vi "appendImage.vi"(8 "error in (no error)":errorcluster, 10 "Image Path":path, 11 "MS-Excel in":refnum<class "MS-Excel.lvclass">) -> (0 "error out":errorcluster, 3 "MS-Excel out":refnum<class "MS-Excel.lvclass">)   [LabVIEW 2017, in "LabVIEW NPOI.lvlib" / "MS-Excel.lvclass"]
uses:
  MS-Excel.lvclass
  MS-Excel.lvclass/MS-Excel.ctl
  C:/Users/Neo/Desktop/Dev_Tools_BR/LabVIEW_NPOI/lib/NPOI 2.1.1/NPOI.dll
  lib/NPOI 2.1.1/NPOI.dll
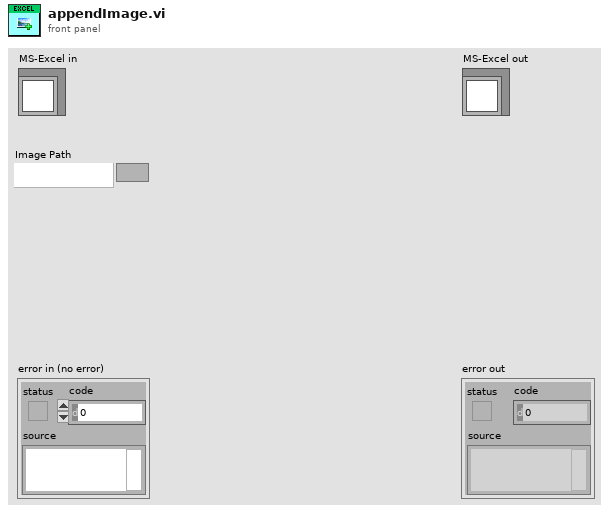
[diagram p1: front panel]
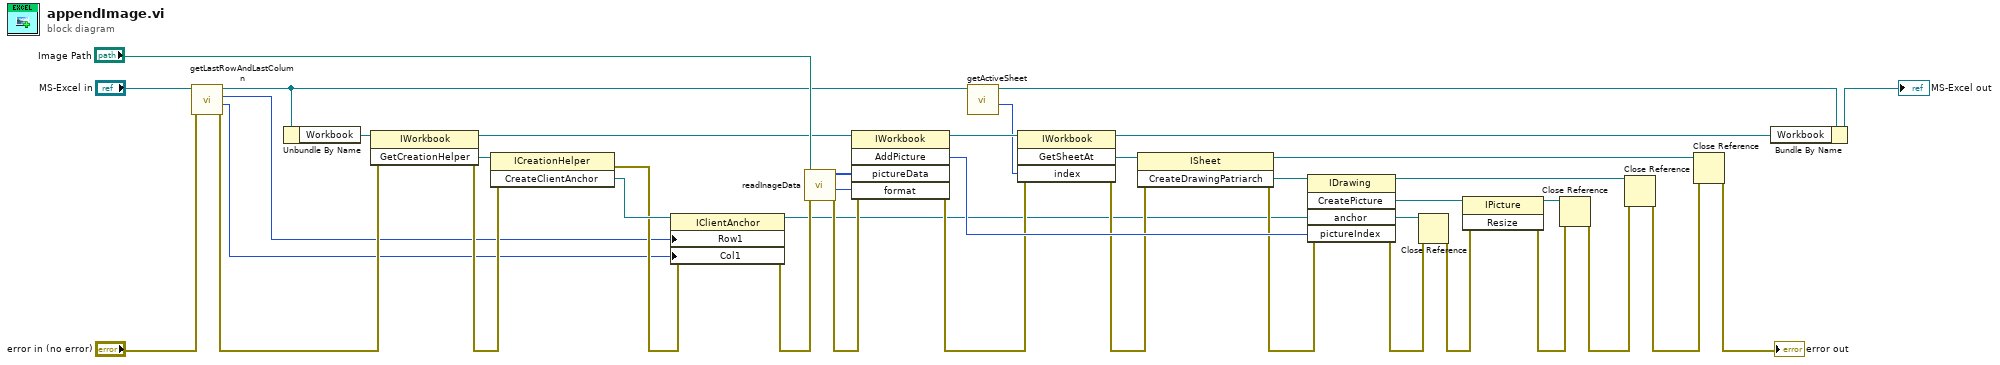
[diagram p0: block diagram]
diagram:
  n1 = call-dynamic "getLastRowAndLastColumn.vi"("error in (no error)"="error in (no error)", "MS-Excel in"="MS-Excel in") -> ("error out"=w23:errorcluster, "Last Column"=w1:i32, "Last Row"=w2:i32, "MS-Excel out"=w26:refnum<class "MS-Excel.lvclass">)  [unwired: 6 in]
  n2 = Unbundle By Name(w26) -> ("Workbook"=w24:refnum<k24>)
  n3 = invoke class="IWorkbook" method="GetCreationHelper"(reference=w24, error in=w23) -> (reference out=w18:refnum<k24>, error out=w22:errorcluster, "GetCreationHelper"=w38:refnum<k24>)  [unwired: 1 in]
  n4 = invoke class="ICreationHelper" method="CreateClientAnchor"(reference=w38, error in=w22) -> (error out=w3:errorcluster, "CreateClientAnchor"=w37:refnum<k24>)  [unwired: 1 in, 1 out]
  n5 = property class="IClientAnchor"(reference=w37, error in=w3, "Row1"=w2, "Col1"=w1) -> (reference out=w16:refnum<k24>, error out=w21:errorcluster)
  n6 = call "readInageData.vi"("error in (no error)"=w21, "file (use dialog)"="Image Path") -> ("error out"=w20:errorcluster, "format"=w28:i32, "Bytes"=w34:u8[])  [unwired: 7 in]
  n7 = invoke class="IWorkbook" method="AddPicture"(reference=w18, error in=w20, "pictureData"=w34, "format"=w28) -> (reference out=w17:refnum<k24>, error out=w19:errorcluster, "AddPicture"=w35:i32)  [unwired: 1 in, 2 out]
  n8 = call-dynamic "getActiveSheet.vi"("MS-Excel in"=w26) -> ("SheetIndex"=w4:i32, "MS-Excel out"=w5:refnum<class "MS-Excel.lvclass">)  [unwired: 7 in, 2 out]
  n9 = invoke class="IWorkbook" method="GetSheetAt"(reference=w17, error in=w19, "index"=w4) -> (reference out=w29:refnum<k24>, error out=w33:errorcluster, "GetSheetAt"=w39:refnum<k24>)  [unwired: 1 in, 1 out]
  n10 = invoke class="ISheet" method="CreateDrawingPatriarch"(reference=w39, error in=w33) -> (reference out=w11:refnum<k24>, error out=w31:errorcluster, "CreateDrawingPatriarch"=w36:refnum<k24>)  [unwired: 1 in]
  n11 = invoke class="IDrawing" method="CreatePicture"(reference=w36, error in=w31, "anchor"=w16, "pictureIndex"=w35) -> (reference out=w12:refnum<k24>, error out=w7:errorcluster, "CreatePicture"=w15:refnum<k24>)  [unwired: 1 in, 2 out]
  n12 = Close Reference(reference=w16, error in (no error)=w7) -> (error out=w8:errorcluster)
  n13 = invoke class="IPicture" method="Resize"(reference=w15, error in=w8) -> (reference out=w14:refnum<k24>, error out=w13:errorcluster)  [unwired: 1 in, 1 out]
  n14 = Close Reference(reference=w14, error in (no error)=w13) -> (error out=w9:errorcluster)
  n15 = Close Reference(reference=w12, error in (no error)=w9) -> (error out=w10:errorcluster)
  n16 = Close Reference(reference=w11, error in (no error)=w10) -> (error out=→"error out":errorcluster)
  n17 = Bundle By Name(cluster=w5, "Workbook"=w29) -> (→"MS-Excel out":refnum<class "MS-Excel.lvclass">)
